vi "ToGraphVizString.vi"(9 "DAG in":refnum<class "DAG.lvclass">) -> (4 "GraphViz string":string)   [LabVIEW 2014, in "DAG.lvclass"]
uses:
  DAG.lvclass
  DAG.lvclass/DAG.ctl
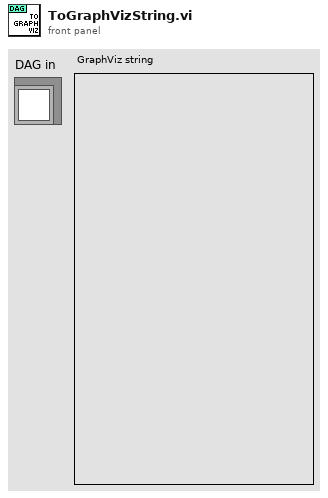
[diagram p1: front panel]
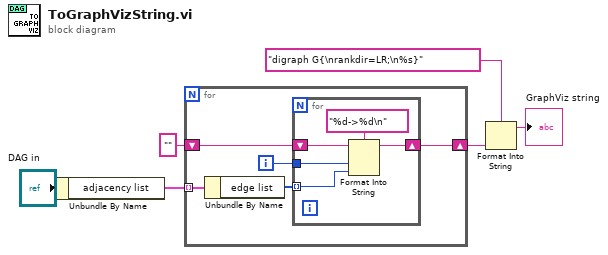
[diagram p0: block diagram]
diagram:
  n1 = Unbundle By Name("DAG in") -> ("adjacency list"=w5:cluster{"edge list":i32[]}[])
  n2 = for {
    tunnel: w5 -> [w11] mode=indexing
    shift-right: [w8] -> w3
    shift-left: "" -> [w7]
    i -> [w9]
    n3 = Unbundle By Name(w11) -> ("edge list"=w10:i32[])
    n4 = for {
      tunnel: w10 -> [w15] mode=indexing
      tunnel: w9 -> [w16]
      shift-right: [w13] -> w8
      shift-left: w7 -> [w12]
      n5 = Format Into String(format string="%d->%d\n", initial string=w12, w16, w15) -> (resulting string=w13:string)  [unwired: 1 in, 1 out]
    }
  }
  n6 = Format Into String(format string="digraph G{\nrankdir=LR;\n%s}", w3) -> (resulting string=→"GraphViz string":string)  [unwired: 2 in, 1 out]
